vi "CenterROI.vi"(0 "object in":refnum<class "Hamamatsu.lvclass">, 5 "error in (no error)":errorcluster) -> (14 "object out":refnum<class "Hamamatsu.lvclass">, 16 "Sub Region":T2 {"V Size"."Value" min=0 max=0 step=4; "H Size"."Value" min=0 max=0 step=4; "V Offset"."Value" min=0 max=0 step=4; "H Offset"."Value" min=0 max=0 step=4}, 19 "error out":errorcluster)   [LabVIEW 2019, in "Hamamatsu.lvclass"]
uses:
  Hamamatsu.lvclass
  <vilib>/Utility/miscctls.llb/LVMinMaxIncTypeDef.ctl
  Hamamatsu.lvclass/Hamamatsu.ctl
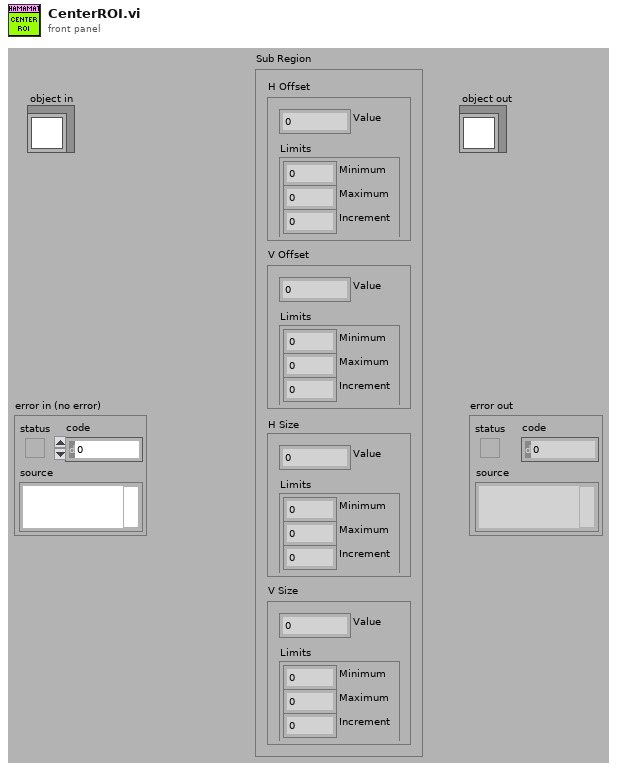
[diagram p1: front panel]
types:
  T1 = typedef "LVMinMaxIncTypeDef.ctl" = cluster{"Minimum":dbl, "Maximum":dbl, "Increment":dbl}
  T2 = cluster{"H Offset":cluster{"Value":i32, "Limits":T1}, "V Offset":cluster{"Value":i32, "Limits":T1}, "H Size":cluster{"Value":i32, "Limits":T1}, "V Size":cluster{"Value":i32, "Limits":T1}}
  T3 = cluster{"Horizontal Offset":i32, "Vertical Offset":i32, "Horizontal Size":i32, "Vertical Size":i32}
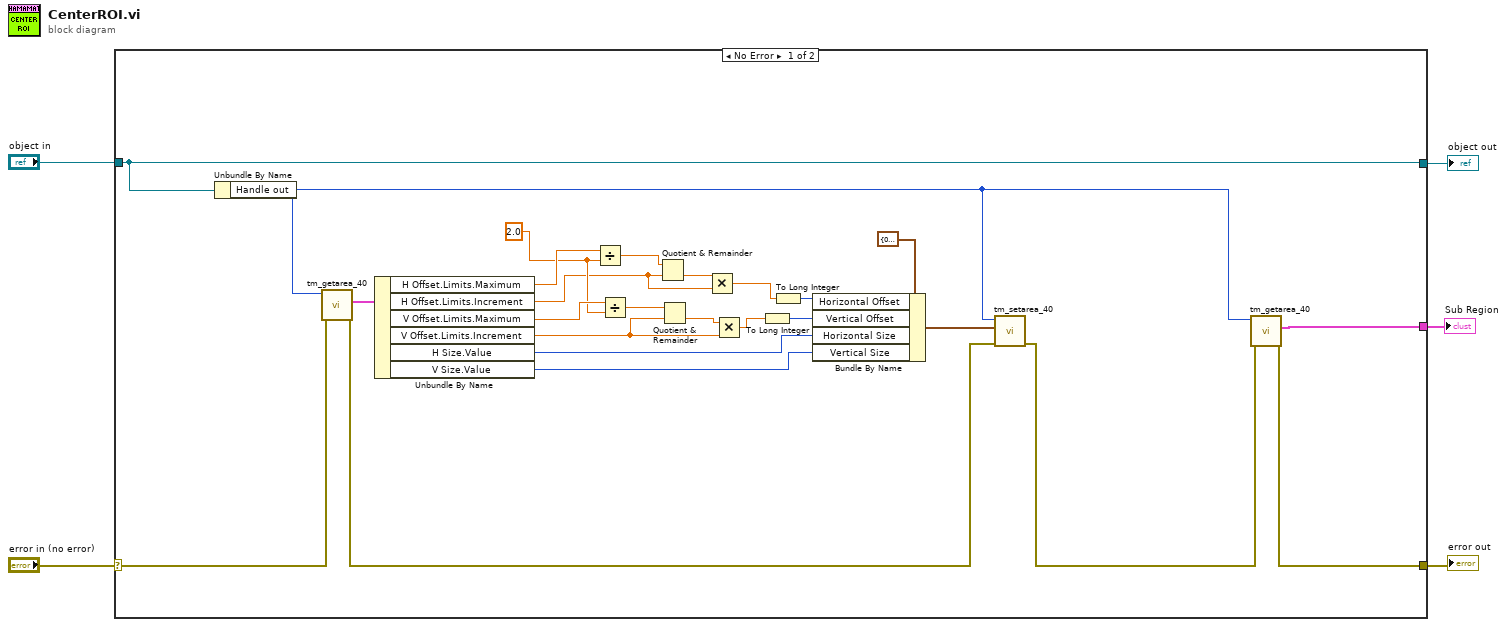
[diagram p0: block diagram]
diagram:
  n1 = case shown="No Error" "error in (no error)" {
    selector: "error in (no error)" -> [w19 w32]
    tunnel: [w22 w32] -> w4
    tunnel: [w21 w31] -> w2
    tunnel: "object in" -> [w21 w31]
    tunnel: [w17 _] -> w1
    frame No Error {
      w13 = 2.0 ("x")
      n2 = Unbundle By Name(w21) -> ("Handle out"=w20:u32)
      n3 = call <userlib>:"tm_getarea_40.vi"("error in (no error)"=w19, "Handle in"=w20) -> ("error out"=w18:errorcluster, "Sub Region"=w30:T2)  [unwired: 7 in, 1 out]
      n4 = Unbundle By Name(w30) -> ("H Offset.Limits.Maximum"=w16:dbl, "H Offset.Limits.Increment"=w11:dbl, "V Offset.Limits.Maximum"=w14:dbl, "V Offset.Limits.Increment"=w8:dbl, "H Size.Value"=w26:i32, "V Size.Value"=w25:i32)
      n5 = Divide(x=w16, y=w13) -> (x/y=w15:dbl)
      n6 = Divide(x=w14, y=w13) -> (x/y=w12:dbl)
      n7 = Quotient & Remainder(x=w15, y=w11) -> (floor(x/y)=w10:dbl)  [unwired: 1 out]
      n8 = Quotient & Remainder(x=w12, y=w8) -> (floor(x/y)=w7:dbl)  [unwired: 1 out]
      n9 = Multiply(x=w10, y=w11) -> (x*y=w9:dbl)
      n10 = Multiply(x=w7, y=w8) -> (x*y=w6:dbl)
      n11 = To Long Integer(number=w6) -> (32bit integer=w27:i32)
      n12 = To Long Integer(number=w9) -> (32bit integer=w28:i32)
      n13 = Bundle By Name(cluster=T3 {"Horizontal Offset"=0, "Vertical Offset"=0, "Horizontal Size"=0, "Vertical Size"=0} ("Sub Region"), "Horizontal Offset"=w28, "Vertical Offset"=w27, "Horizontal Size"=w26, "Vertical Size"=w25) -> (w24:T3)
      n14 = call <userlib>:"tm_setarea_40.vi"("error in (no error)"=w18, "Sub Region"=w24, "Handle in"=w20) -> ("error out"=w23:errorcluster)  [unwired: 7 in, 1 out]
      n15 = call <userlib>:"tm_getarea_40.vi"("error in (no error)"=w23, "Handle in"=w20) -> ("error out"=w22:errorcluster, "Sub Region"=w17:T2)  [unwired: 7 in, 1 out]
    }
    frame Error {
    }
  }
  "error out" <- w4
  "object out" <- w2
  "Sub Region" <- w1
